vi "Error Query (multiple).vi"(0 "VISA resource name":refnum<visa-resource-name>, 11 "error in (no error)":errorcluster) -> (4 "VISA resource name out":refnum<visa-resource-name>, 8 "Error":i32[](array[numeric]), 10 "Error Message":string, 15 "error out":errorcluster)   [LabVIEW 2013, in "Yokogawa WT200 Series.lvlib"]
doc: "This VI reads the error queue from the instrument. It expects to see errors in SCPI format (#,\"error message\"). It continues to read from the error queue until it reads a 0, \"No error\"."
uses:
  <instrlib>/Yokogawa WT200 Series/Yokogawa WT200 Series.lvlib
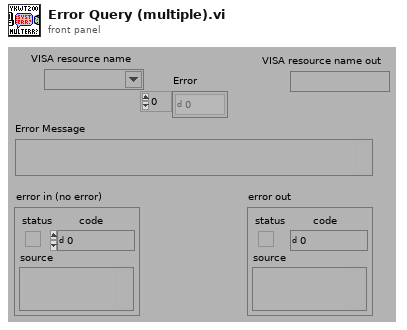
[diagram p1: front panel]
types:
  T1 = cluster{"Status":bool, "Error":i32, "source":string}
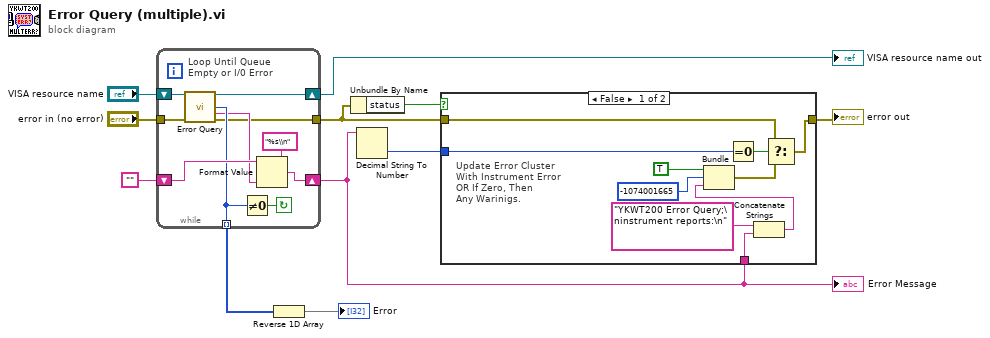
[diagram p0: block diagram]
diagram:
  n1 = while {
    tunnel: "error in (no error)" -> [w15]
    tunnel: [w14] -> w2 mode=indexing
    tunnel: [w12] -> w11
    shift-left: "VISA resource name" -> [w16]
    shift-right: [w21] -> w5
    shift-left: "" -> [w18]
    shift-right: [w20] -> w3
    stop <- w17 continue-if-true
    # "Loop Until Queue Empty or I/0 Error"
    n2 = call <instrlib>:"Error Query.vi"("VISA resource name"=w16, "error in (no error)"=w15) -> ("VISA resource name out"=w21:refnum<visa-resource-name>, "Error"=w14:i32, "Error Message"=w13:string, "error out"=w12:errorcluster)  [unwired: 10 in]
    n3 = Not Equal To 0?(x=w14) -> (x != 0?=w17:bool)
    n4 = Format Value(string ("")=w18, format string="%s\\n", value (0)=w13) -> (output string=w20:string)
  }
  "Error Message" <- w3
  "VISA resource name out" <- w5
  n5 = Reverse 1D Array(array=w2) -> (reversed array=→"Error":i32[])
  n6 = Unbundle By Name(w11) -> ("status"=w10:bool)
  n7 = Decimal String To Number(string=w3) -> (number=w9:i32)  [unwired: 2 in, 1 out]
  n8 = case shown="False" w10 {
    tunnel: w9 -> [w22 _]
    tunnel: [w25 w32] -> w4
    tunnel: w11 -> [w24 w32]
    tunnel: w3 -> [w31 _]
    frame False {
      # "Update Error Cluster\nWith Instrument Error \nOR If Zero, Then \nAny Warinigs."
      n9 = Equal To 0?(x=w22) -> (x = 0?=w26:bool)
      n10 = Concatenate Strings("YKWT200 Error Query;\ninstrument reports:\n" ("Source"), w31) -> (w28:string)
      n11 = Bundle("Status"=TRUE, "Error"=-1074001665, w28) -> (w23:cluster{"Status":bool, "Error":i32, string})  [unwired: 1 in]
      n12 = Select(t=w24, s=w26, f=w23) -> (s? t:f=w25:T1)
    }
    frame True {
      # "IO Error"
    }
  }
  "error out" <- w4
